vi "GET_PRESTATUS.vi"(10 "CODE_ID":string, 11 "PRODUCT_ID":string) -> (2 "字符串":string, 3 "OK?":bool)   [LabVIEW 2020]
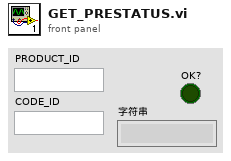
[diagram p1: front panel]
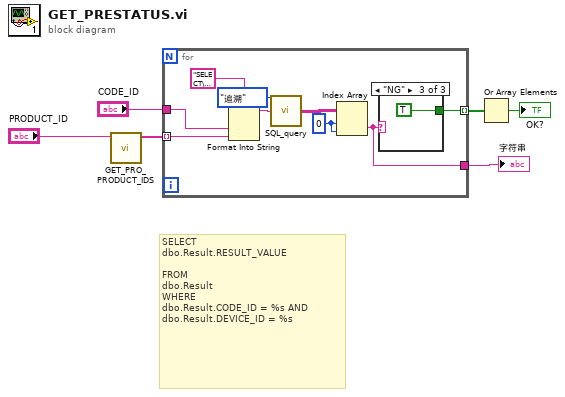
[diagram p0: block diagram]
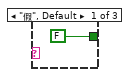
[diagram p2: hidden frame]
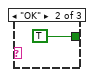
[diagram p3: hidden frame]
diagram:
  # "SELECT\ndbo.Result.RESULT_VALUE\n\nFROM\ndbo.Result\nWHERE\ndbo.Result.CODE_ID = %s AND\ndbo.Result.DEVICE_ID = %s"
  n1 = call "GET_PRO_PRODUCT_IDS.vi"("PRODUCT_ID"="PRODUCT_ID") -> ("前序工位"=w5:string[])  [unwired: 10 in]
  n2 = for {
    tunnel: w5 -> [w14] mode=indexing
    tunnel: "CODE_ID" -> [w13]
    tunnel: [w9] -> w3 mode=indexing
    tunnel: [w8] -> w1
    w10 = 0 ("索引 (行)")
    n3 = Format Into String(format string="SELECT\ndbo.Result.RESULT_VALUE\n\nFROM\ndbo.Result\nWHERE\ndbo.Result.CODE_ID = %s AND\ndbo.Result.DEVICE_ID = %s\n" ("格式字符串"), w13, w14) -> (resulting string=w12:string)  [unwired: 2 in, 1 out]
    n4 = call "SQL_query.vi"("SQL query"=w12, "联机模式"=enum16{"单机", "追溯"}."追溯") -> ("data"=w11:string[][])  [unwired: 2 in, 1 out]
    n5 = Index Array(array=w11, index (row)=w10, index (col)=w10) -> (element=w8:string)
    n6 = case shown="\"NG\"" w8 {
      tunnel: [FALSE TRUE TRUE] -> w9
      frame "假", Default {
      }
      frame "OK" {
      }
      frame "NG" {
      }
    }
  }
  "字符串" <- w1
  n7 = Or Array Elements(Boolean array=w3) -> (logical OR=→"OK?":bool)
